vi "GPIO Bank Crosspoint Switch.vi"(0 "source gpio bank in":T2, 5 "source user gpio in":bool, 7 "destination user gpio in":bool, 11 "gpio bank routing":i32[](array[numeric])=[-1, -1, -1, -1, -1, -1, -1, -1, -1, -1, -1, -1]) -> (4 "destination gpio bank output config":T1, 8 "destination user gpio out":bool)   [LabVIEW 2020, in "GettingStarted_Common_148X_FPGA.lvlib"]
uses:
  GettingStarted_Common_148X_FPGA.lvlib
  <instrlib>/FlexRIO/CSI-2/v2/FPGA/Types/GPIO Bank.ctl
  Types/GPIO Bank Output Configuration.ctl
  <instrlib>/FlexRIO/CSI-2/v2/FPGA/NI CSI-2 API FPGA v2.lvlib
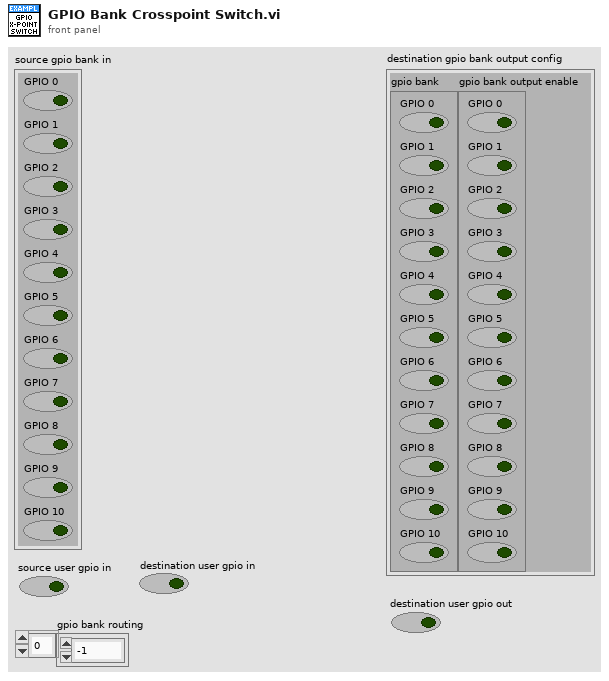
[diagram p1: front panel]
types:
  T1 = typedef "GettingStarted_Common_148X_FPGA.lvlib/GPIO Bank Output Configuration.ctl" = cluster{"gpio bank":T2, "gpio bank output enable":T2}
  T2 = typedef "NI CSI-2 API FPGA v2.lvlib/GPIO Bank.ctl" = cluster{"GPIO 0":bool, "GPIO 1":bool, "GPIO 2":bool, "GPIO 3":bool, "GPIO 4":bool, "GPIO 5":bool, "GPIO 6":bool, "GPIO 7":bool, "GPIO 8":bool, "GPIO 9":bool, "GPIO 10":bool}
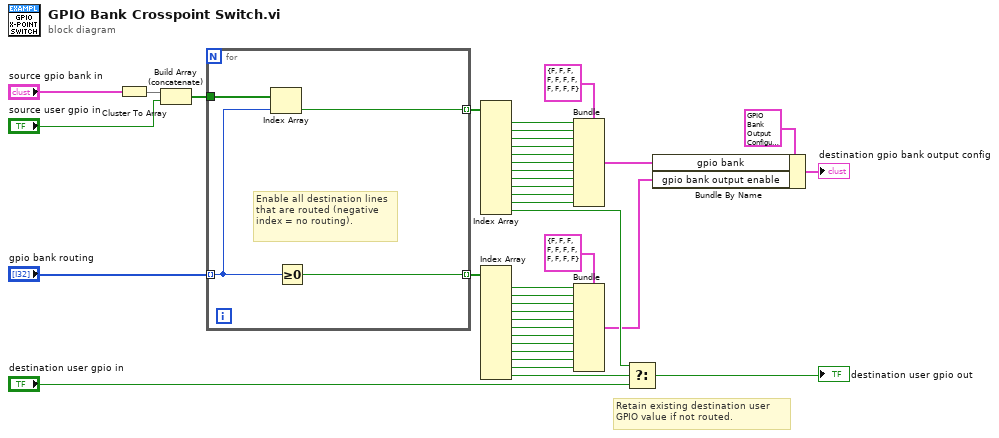
[diagram p0: block diagram]
diagram:
  # "Retain existing destination user GPIO value if not routed."
  n1 = Cluster To Array(cluster="source gpio bank in") -> (array=w25:bool[])
  n2 = Build Array (concatenate)(w25, "source user gpio in") -> (w24:bool[])
  n3 = for {
    tunnel: w24 -> [w43]
    tunnel: "gpio bank routing" -> [w42] mode=indexing
    tunnel: [w41] -> w10 mode=indexing
    tunnel: [w40] -> w9 mode=indexing
    # "Enable all destination lines that are routed (negative index = no routing)."
    n4 = Index Array(array=w43, index=w42) -> (element=w40:bool)
    n5 = Greater Or Equal To 0?(x=w42) -> (x >= 0?=w41:bool)
  }
  n6 = Index Array(array=w9) -> (element #1=w29:bool, element #2=w30:bool, element #3=w31:bool, element #4=w32:bool, element #5=w33:bool, element #6=w34:bool, element #7=w35:bool, element #8=w36:bool, element #9=w37:bool, element #10=w38:bool, element #11=w39:bool, element #12=w6:bool)  [unwired: 12 in]
  n7 = Index Array(array=w10) -> (element #1=w21:bool, element #2=w20:bool, element #3=w19:bool, element #4=w18:bool, element #5=w17:bool, element #6=w16:bool, element #7=w15:bool, element #8=w14:bool, element #9=w13:bool, element #10=w12:bool, element #11=w11:bool, element #12=w8:bool)  [unwired: 12 in]
  n8 = Bundle(cluster=T2 {"GPIO 0"=FALSE, "GPIO 1"=FALSE, "GPIO 2"=FALSE, "GPIO 3"=FALSE, "GPIO 4"=FALSE, "GPIO 5"=FALSE, "GPIO 6"=FALSE, "GPIO 7"=FALSE, "GPIO 8"=FALSE, "GPIO 9"=FALSE, "GPIO 10"=FALSE} ("gpio bank output"), "GPIO 0"=w29, "GPIO 1"=w30, "GPIO 2"=w31, "GPIO 3"=w32, "GPIO 4"=w33, "GPIO 5"=w34, "GPIO 6"=w35, "GPIO 7"=w36, "GPIO 8"=w37, "GPIO 9"=w38, "GPIO 10"=w39) -> (w4:T2)
  n9 = Bundle(cluster=T2 {"GPIO 0"=FALSE, "GPIO 1"=FALSE, "GPIO 2"=FALSE, "GPIO 3"=FALSE, "GPIO 4"=FALSE, "GPIO 5"=FALSE, "GPIO 6"=FALSE, "GPIO 7"=FALSE, "GPIO 8"=FALSE, "GPIO 9"=FALSE, "GPIO 10"=FALSE} ("gpio bank output"), "GPIO 0"=w21, "GPIO 1"=w20, "GPIO 2"=w19, "GPIO 3"=w18, "GPIO 4"=w17, "GPIO 5"=w16, "GPIO 6"=w15, "GPIO 7"=w14, "GPIO 8"=w13, "GPIO 9"=w12, "GPIO 10"=w11) -> (w3:T2)
  n10 = Select(t=w6, s=w8, f="destination user gpio in") -> (s? t:f=→"destination user gpio out":bool)
  n11 = Bundle By Name(cluster=T1 {"gpio bank"={"GPIO 0"=FALSE, "GPIO 1"=FALSE, "GPIO 2"=FALSE, "GPIO 3"=FALSE, "GPIO 4"=FALSE, "GPIO 5"=FALSE, "GPIO 6"=FALSE, "GPIO 7"=FALSE, "GPIO 8"=FALSE, "GPIO 9"=FALSE, "GPIO 10"=FALSE}, "gpio bank output enable"={"GPIO 0"=FALSE, "GPIO 1"=FALSE, "GPIO 2"=FALSE, "GPIO 3"=FALSE, "GPIO 4"=FALSE, "GPIO 5"=FALSE, "GPIO 6"=FALSE, "GPIO 7"=FALSE, "GPIO 8"=FALSE, "GPIO 9"=FALSE, "GPIO 10"=FALSE}} ("destination gpio bank output config"), "gpio bank"=w4, "gpio bank output enable"=w3) -> (→"destination gpio bank output config":T1)
